vi "Create.vi"(9 "Alias":string, 10 "Queue Actor":refnum<class "Queue Actor.lvclass">, 11 "Dev Actor in":refnum<class "Dev Actor.lvclass">) -> (3 "Dev Actor out":refnum<class "Dev Actor.lvclass">)   [LabVIEW 2021, in "Dev Actor.lvlib" / "Dev Actor.lvclass"]
uses:
  Dev Actor.lvclass
  Queue Actor/Queue Actor.lvclass
  Dev Actor.lvclass/Dev Actor.ctl
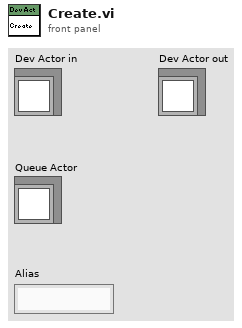
[diagram p1: front panel]
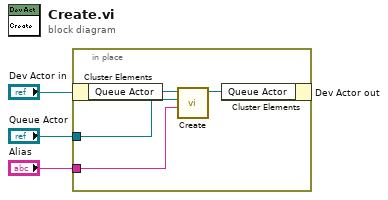
[diagram p0: block diagram]
diagram:
  n1 = in-place {
    in-place-border: "Queue Actor" -> [w5]
    in-place-border: "Alias" -> [w6]
    n2 = in-place-cluster #1("Dev Actor in") -> ("Queue Actor"=w7:refnum<class "Queue Actor.lvclass">)
    n3 = call-dynamic "Create.vi"("Alias"=w6, "Queue Actor"=w5, "Create in"=w7) -> ("Create out"=w8:refnum<class "Queue Actor.lvclass">)  [unwired: 8 in]
    n4 = in-place-cluster #1("Queue Actor"=w8) -> (→"Dev Actor out":refnum<class "Dev Actor.lvclass">)
  }
